vi "Pause.vi"(8 "error in (no error)":errorcluster, 10 "Internal?":bool, 11 "Huber Settings In":T1) -> (0 "error out":errorcluster, 3 "Huber Settings Out":T1)   [LabVIEW 2018, in "Huber Unistat 410 TCU.lvlib"]
uses:
  Huber Unistat 410 TCU.lvlib
  Huber Unistat 410 Settings.ctl
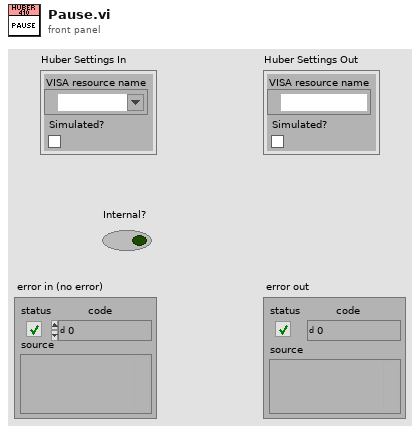
[diagram p1: front panel]
types:
  T1 = typedef "Huber Unistat 410 TCU.lvlib/Huber Unistat 410 Settings.ctl" = cluster{"VISA resource name":refnum<visa-resource-name>, "Simulated?":bool}
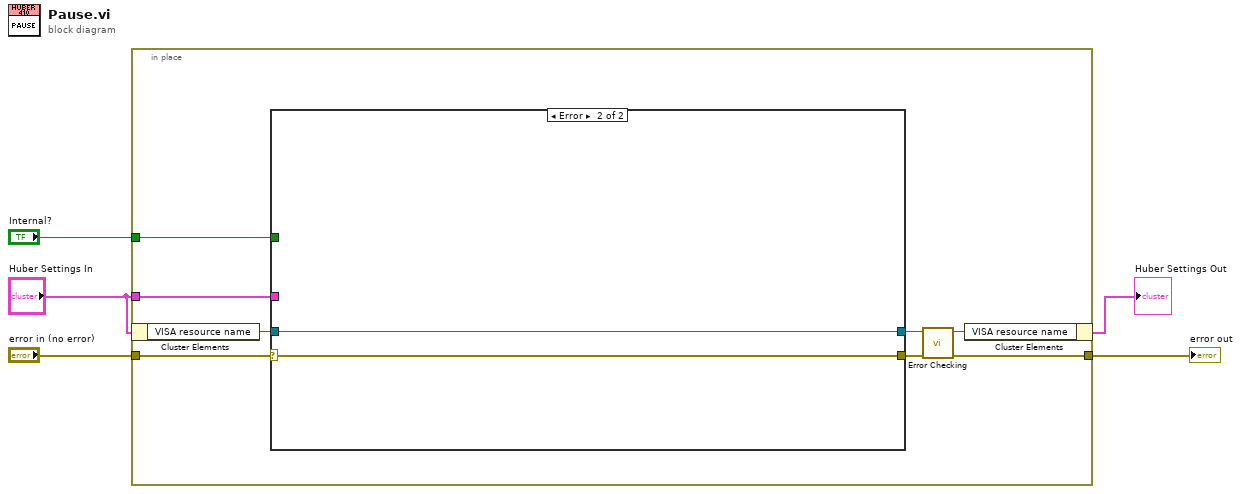
[diagram p0: block diagram]
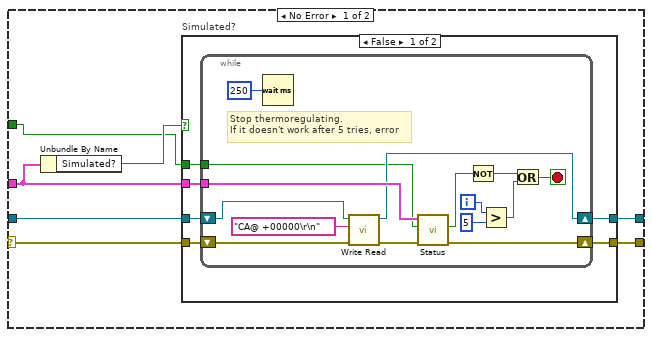
[diagram p2: hidden frame]
diagram:
  n1 = in-place {
    in-place-border: "error in (no error)" -> [w13]
    in-place-border: [w10] -> w4
    in-place-border: "Huber Settings In" -> [w9]
    in-place-border: "Internal?" -> [w8]
    n2 = in-place-cluster #1("Huber Settings In") -> ("VISA resource name"=w7:refnum<visa-resource-name>)
    n3 = case shown="Error" w13 {
      selector: w13 -> [w20 w45]
      tunnel: w9 -> [w16 _]
      tunnel: [w19 w45] -> w11
      tunnel: [w18 w44] -> w12
      tunnel: w8 -> [w15 _]
      tunnel: w7 -> [w14 w44]
      frame No Error {
        n4 = Unbundle By Name(w16) -> ("Simulated?"=w17:bool)
        n5 = case "Simulated?" shown="False" w17 {
          tunnel: w20 -> [w24 w43]
          tunnel: [w22 w43] -> w19
          tunnel: [w26 w42] -> w18
          tunnel: w14 -> [w25 w42]
          tunnel: w16 -> [w23 _]
          tunnel: w15 -> [w21 _]
          frame False {
            n6 = while {
              tunnel: w23 -> [w41]
              shift-right: [w31] -> w26
              shift-left: w25 -> [w34]
              shift-right: [w40] -> w22
              shift-left: w24 -> [w32]
              tunnel: w21 -> [w27]
              i -> [w38]
              stop <- w39 stop-if-true
              # "Stop thermoregulating. \nIf it doesn't work after 5 tries, error"
              n7 = Wait (ms)(milliseconds to wait=u32 250) -> ()  [unwired: 1 out]
              n8 = call "Write Read.vi"("error in (no error)"=w32, "write string"="CA@ +00000\r\n" ("string"), "VISA Refnum in"=w34) -> ("error out"=w30:errorcluster, "VISA Refnum out"=w31:refnum<visa-resource-name>)  [unwired: 6 in, 1 out]
              n9 = call "Status.vi"("error in (no error)"=w30, "Internal?"=w27, "Huber Settings In"=w41) -> ("error out"=w40:errorcluster, "Running"=w29:bool)  [unwired: 4 in, 3 out]
              n10 = Not(x=w29) -> (.not. x?=w28:bool)
              n11 = Greater?(x=w38, y=5) -> (0:w36:bool)
              n12 = Or(x=w28, y=w36) -> (x .or. y?=w39:bool)
            }
          }
          frame True {
          }
        }
      }
      frame Error {
      }
    }
    n13 = call "Error Checking.vi"("error in (no error)"=w11, "VISA resource name"=w12) -> ("error out"=w10:errorcluster, "VISA resource name"=w6:refnum<visa-resource-name>)  [unwired: 7 in, 1 out]
    n14 = in-place-cluster #1("VISA resource name"=w6) -> (→"Huber Settings Out":T1)
  }
  "error out" <- w4
